vi "CreateSocket.vi"() -> ()   [LabVIEW 2021]
panel:
  in  "connection in":string="dstp://localhost/aaa"
  in  "Stop Button":bool
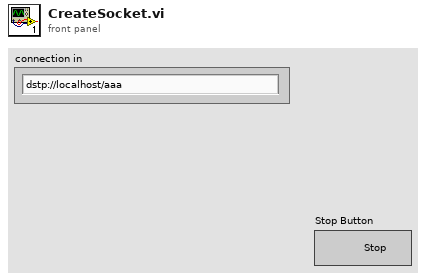
[diagram p1: front panel]
types:
  T1 = enum16{"Read", "Write", "ReadWrite", "BufferedRead", "BufferedReadWrite"}
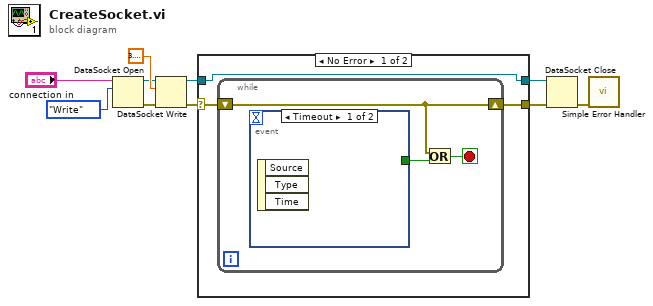
[diagram p0: block diagram]
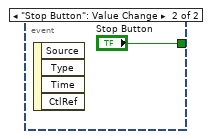
[diagram p2: hidden frame]
diagram:
  n1 = DataSocket Open(10:T1."Write" ("mode"), 11:"connection in") -> (0:w8:errorcluster, 3:w6:refnum<k13>)  [unwired: 2 in]
  n2 = DataSocket Write(8:w8, 10:3.141592653589793, 11:w6) -> (0:w9:errorcluster, 3:w1:refnum<k13>)  [unwired: 1 in, 1 out]
  n3 = case shown="No Error" w9 {
    selector: w9 -> [w12 w19]
    tunnel: [w13 w19] -> w4
    tunnel: [w11 w18] -> w2
    tunnel: w1 -> [w11 w18]
    frame No Error {
      n4 = while {
        shift-right: [w14] -> w13
        shift-left: w12 -> [w14]
        stop <- w15 stop-if-true
        n5 = event shown="[0] Timeout" {
          selector: _ -> [_ _]
          dyn-events: _ -> [_ _]
          timeout: _ -> [_ _]
          tunnel: [_ "Stop Button"] -> w16
          event Timeout {
            n6 = event-data() -> ()  [unwired: 1 in, 3 out]
          }
          event "Stop Button": Value Change {
            n7 = event-data() -> ()  [unwired: 1 in, 4 out]
          }
        }
        n8 = Or(x=w14, y=w16) -> (x .or. y?=w15:bool)
      }
    }
    frame Error {
    }
  }
  n9 = DataSocket Close(8:w4, 11:w2) -> (0:w3:errorcluster)  [unwired: 1 in, 1 out]
  n10 = call <vilib>:"Simple Error Handler.vi"("error in (no error)"=w3) -> ()  [unwired: 4 in, 5 out]
